vi "SetUp.vi"(8 "error in (no error)":errorcluster, 11 "Prueba21 in":refnum<class "Prueba21.lvclass">) -> (0 "error out":errorcluster, 3 "Prueba21 out":refnum<class "Prueba21.lvclass">)   [LabVIEW 2019, in "Prueba21.lvclass"]
uses:
  Prueba21.lvclass
  Prueba21.lvclass/Prueba21.ctl
  Prueba/Prueba.lvclass
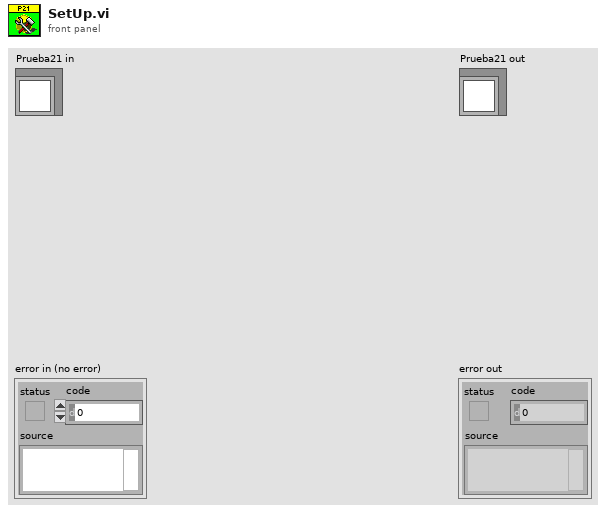
[diagram p1: front panel]
types:
  T1 = typedef "Prueba21.lvclass/BD.ctl" = cluster{"Frec_Referencia":dbl, "IncertidumbreNPS":string[], "Tol_Abs_dB":string[], "IncertidumbreFrec":string[], "Tol_Abs_Hz":string[], "IncertidumbreTD":string[], "MaxTol%":string[]}
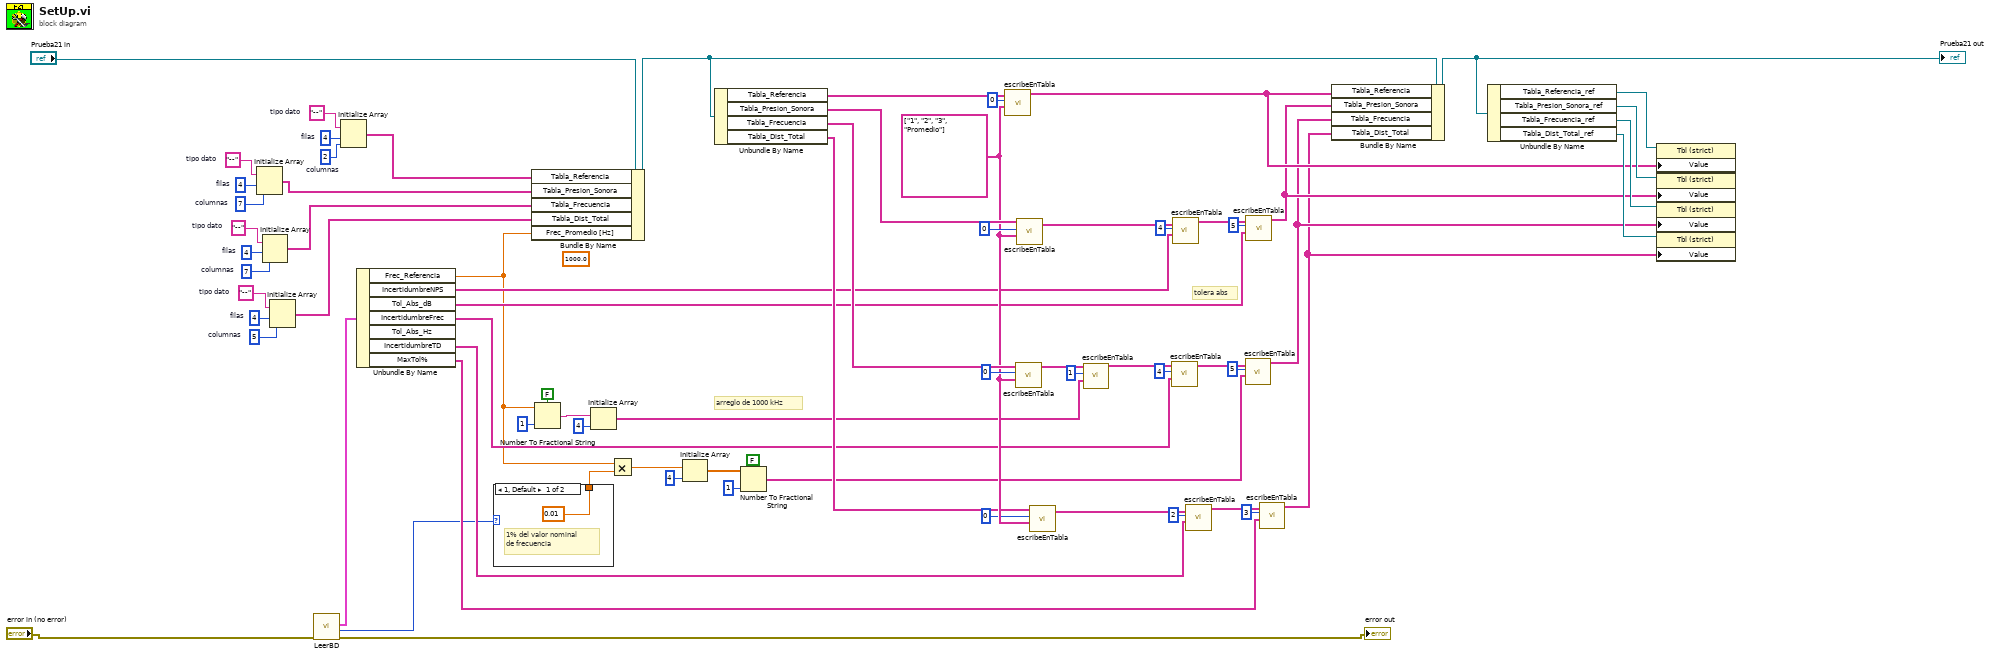
[diagram p0: block diagram]
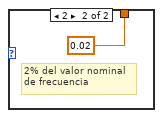
[diagram p2: hidden frame]
diagram:
  (unwired) 1000.0 ("Frec_Promedio [Hz]")
  w38 = string[] ["1", "2", "3", "Promedio"]
  w59 = 5  # columnas
  w58 = 4  # filas
  w60 = "--"  # tipo dato
  w63 = 7  # columnas
  w64 = 4  # filas
  w61 = "--"  # tipo dato
  w65 = 2  # columnas
  w66 = 4  # filas
  w68 = "--"  # tipo dato
  w71 = 7  # columnas
  w69 = 4  # filas
  w72 = "--"  # tipo dato
  # "arreglo de 1000 kHz"
  # "tolera abs"
  n1 = Initialize Array(w72, w69, w71) -> (w70:string[][])
  n2 = Initialize Array(w61, w64, w63) -> (w62:string[][])
  n3 = Initialize Array(w60, w58, w59) -> (w57:string[][])
  n4 = call "LeerBD.vi"("error in (no error)"="error in (no error)") -> ("error out"=→"error out":errorcluster, "clase"=w6:i32, "BD"=w24:T1)  [unwired: 8 in]
  n5 = Initialize Array(w68, w66, w65) -> (w67:string[][])
  n6 = Unbundle By Name(w24) -> ("Frec_Referencia"=w8:dbl, "IncertidumbreNPS"=w18:string[], "Tol_Abs_dB"=w12:string[], "IncertidumbreFrec"=w11:string[], "IncertidumbreTD"=w9:string[], "MaxTol%"=w7:string[])  [unwired: 1 out]
  n7 = case shown="1, Default" w6 {
    tunnel: [0.01 ("y") 0.02 ("y")] -> w17
    frame 1, Default {
      # "1% del valor nominal\nde frecuencia"
    }
    frame 2 {
      # "2% del valor nominal\nde frecuencia"
    }
  }
  n8 = Bundle By Name(cluster="Prueba21 in", "Tabla_Referencia"=w67, "Tabla_Presion_Sonora"=w70, "Tabla_Frecuencia"=w62, "Tabla_Dist_Total"=w57, "Frec_Promedio [Hz]"=w8) -> (w56:refnum<class "Prueba21.lvclass">)
  n9 = Number To Fractional String(use system decimal point (T)=FALSE, number=w8, precision (6)=i16 1) -> (F-format string=w21:string)  [unwired: 1 in]
  n10 = Initialize Array(w21, 4 ("dimension size")) -> (w19:string[])
  n11 = Multiply(x=w8, y=w17) -> (x*y=w15:dbl)
  n12 = Initialize Array(w15, 4 ("dimension size")) -> (w14:dbl[])
  n13 = Unbundle By Name(w56) -> ("Tabla_Referencia"=w54:string[][], "Tabla_Presion_Sonora"=w52:string[][], "Tabla_Frecuencia"=w43:string[][], "Tabla_Dist_Total"=w36:string[][])
  n14 = Number To Fractional String(use system decimal point (T)=FALSE, number=w14, precision (6)=i16 1) -> (F-format string=w10:string[])  [unwired: 1 in]
  n15 = call "escribeEnTabla.vi"("parametros"=w38, "col"=0, "tabla in"=w54) -> ("tabla out"=w31:string[][])  [unwired: 8 in]
  n16 = call "escribeEnTabla.vi"("parametros"=w38, "col"=0, "tabla in"=w43) -> ("tabla out"=w27:string[][])  [unwired: 8 in]
  n17 = call "escribeEnTabla.vi"("parametros"=w38, "col"=0, "tabla in"=w52) -> ("tabla out"=w51:string[][])  [unwired: 8 in]
  n18 = call "escribeEnTabla.vi"("parametros"=w38, "col"=0, "tabla in"=w36) -> ("tabla out"=w42:string[][])  [unwired: 8 in]
  n19 = call "escribeEnTabla.vi"("parametros"=w19, "col"=1, "tabla in"=w27) -> ("tabla out"=w26:string[][])  [unwired: 8 in]
  n20 = call "escribeEnTabla.vi"("parametros"=w11, "col"=4, "tabla in"=w26) -> ("tabla out"=w47:string[][])  [unwired: 8 in]
  n21 = call "escribeEnTabla.vi"("parametros"=w18, "col"=4, "tabla in"=w51) -> ("tabla out"=w48:string[][])  [unwired: 8 in]
  n22 = call "escribeEnTabla.vi"("parametros"=w9, "col"=2, "tabla in"=w42) -> ("tabla out"=w39:string[][])  [unwired: 8 in]
  n23 = call "escribeEnTabla.vi"("parametros"=w10, "col"=5, "tabla in"=w47) -> ("tabla out"=w29:string[][])  [unwired: 8 in]
  n24 = call "escribeEnTabla.vi"("parametros"=w12, "col"=5, "tabla in"=w48) -> ("tabla out"=w30:string[][])  [unwired: 8 in]
  n25 = call "escribeEnTabla.vi"("parametros"=w7, "col"=3, "tabla in"=w39) -> ("tabla out"=w28:string[][])  [unwired: 8 in]
  n26 = Bundle By Name(cluster=w56, "Tabla_Referencia"=w31, "Tabla_Presion_Sonora"=w30, "Tabla_Frecuencia"=w29, "Tabla_Dist_Total"=w28) -> (w1:refnum<class "Prueba21.lvclass">)
  "Prueba21 out" <- w1
  n27 = Unbundle By Name(w1) -> ("Tabla_Referencia_ref"=w35:refnum<vi>, "Tabla_Presion_Sonora_ref"=w34:refnum<vi>, "Tabla_Frecuencia_ref"=w33:refnum<vi>, "Tabla_Dist_Total_ref"=w32:refnum<vi>)
  n28 = property class="Tbl (strict)"(reference=w35, "Value"=w31) -> ()  [unwired: 1 in, 2 out]
  n29 = property class="Tbl (strict)"(reference=w34, "Value"=w30) -> ()  [unwired: 1 in, 2 out]
  n30 = property class="Tbl (strict)"(reference=w33, "Value"=w29) -> ()  [unwired: 1 in, 2 out]
  n31 = property class="Tbl (strict)"(reference=w32, "Value"=w28) -> ()  [unwired: 1 in, 2 out]
